vi "Process VIA.vi"(8 "error in (no error)":errorcluster, 10 "Raw VIA":string, 11 "RP2040.lvlib:RP2040Platform in":refnum<class "RP2040Platform.lvclass">) -> (0 "error out":errorcluster, 2 "VIA":string, 3 "RP2040.lvlib:RP2040Platform out":refnum<class "RP2040Platform.lvclass">)   [LabVIEW 2020, in "RP2040.lvlib" / "RP2040Platform.lvclass"]
uses:
  RP2040Platform.lvclass
  Builds/picoG/ppl/PicoG-Core.lvlibp/PicoG-Processor/PicoG-Core/DeployPlatform/DeployPlatform.lvclass
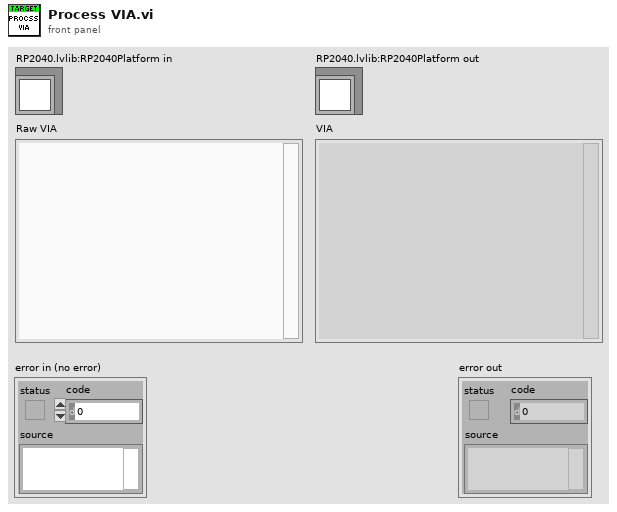
[diagram p1: front panel]
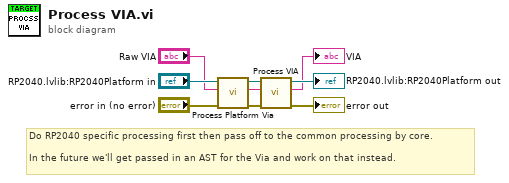
[diagram p0: block diagram]
diagram:
  # "Do RP2040 specific processing first then pass off to the common processing by core.\n\nIn the future we'll get passed in an AST for the Via and work on that instead."
  n1 = call "Process Platform Via.vi"("error in (no error)"="error in (no error)", "Raw VIA"="Raw VIA", "RP2040Platform in"="RP2040.lvlib:RP2040Platform in") -> ("error out"=w5:errorcluster, "VIA"=w3:string, "RP2040Platform out"=w4:refnum<class "RP2040Platform.lvclass">)  [unwired: 6 in]
  n2 = call-parent "Process VIA.vi"("error in (no error)"=w5, "Raw VIA"=w3, "DeployTarget in"=w4) -> ("error out"=→"error out":errorcluster, "VIA"=→"VIA":string, "DeployTarget out"=→"RP2040.lvlib:RP2040Platform out":refnum<class "RP2040Platform.lvclass">)  [unwired: 6 in]
